vi "yzk3.4.vi"(2 "字符串 3":string, 3 "字符串 2":string, 4 "字符串":string) -> (0 "长度":i32, 1 "连接的字符串":string)   [LabVIEW 2017]
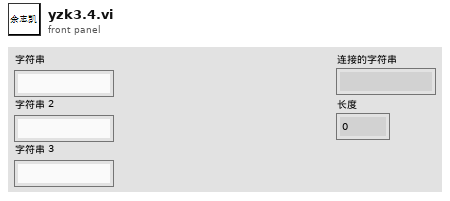
[diagram p1: front panel]
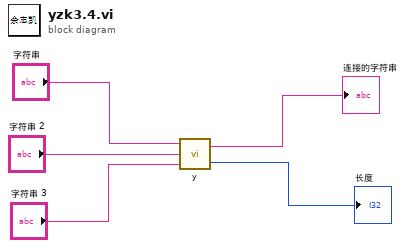
[diagram p0: block diagram]
diagram:
  n1 = call "y.vi"("字符串 3"="字符串 3", "字符串 2"="字符串 2", "字符串"="字符串") -> ("长度"=→"长度":i32, "连接的字符串"=→"连接的字符串":string)
